vi "step_HAPS_Compressor_worksheet.vi"() -> ()   [LabVIEW 2020]
uses:
  <vilib>/AKKA/PROVEtech-RBS/PROVEtechRBS.lvlib
  <vilib>/AKKA/PROVEtech-RBS/SubVIs/Write (Signals Single-point).vi
  <vilib>/AKKA/PROVEtech-RBS/SubVIs/Read (Signals Single-point).vi
panel:
  out "receive unit":string[](array[string])
  out "pass":bool
  out "Array out":string[](array[string])
  out "receive signals":string[](array[string])
  out "sgl array":dbl[](array[numeric])
  out "send unit":string[](array[string])
  out "send values":string[](array[string])
  out "send signals":string[](array[string])
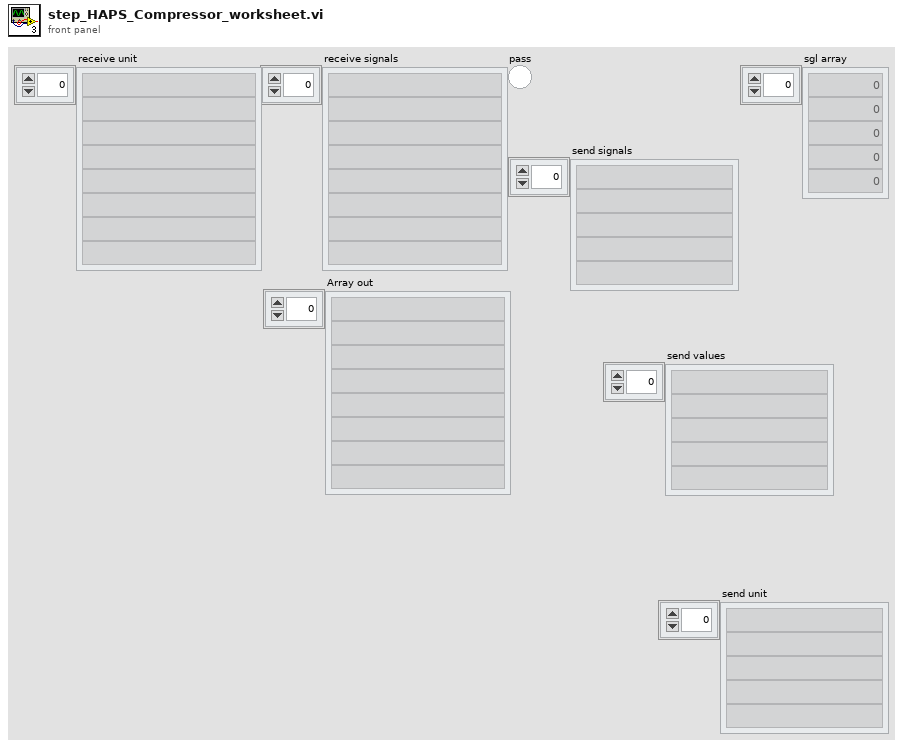
[diagram p1: front panel]
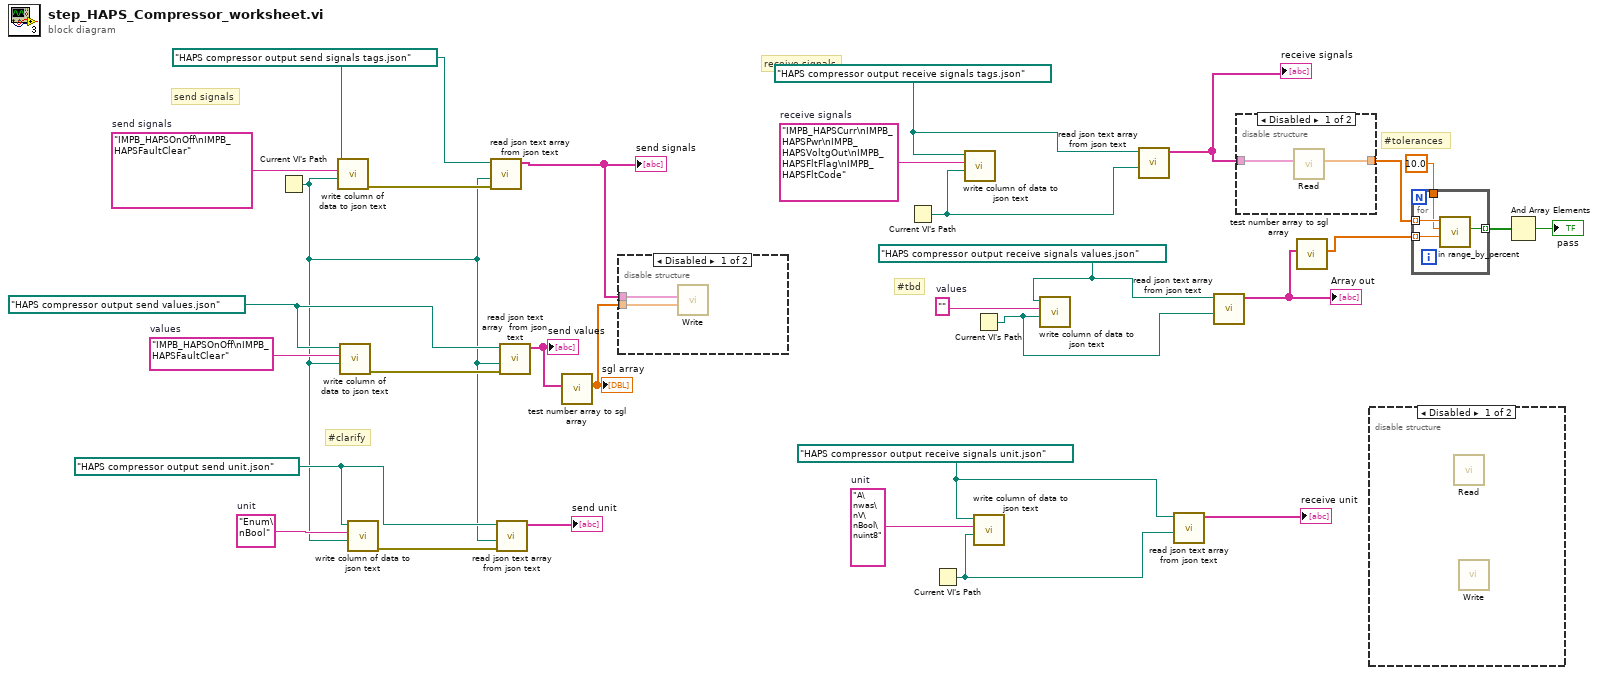
[diagram p0: block diagram]
diagram:
  w3 = path "HAPS compressor output receive signals unit.json" ("name or relative path")
  w13 = path "HAPS compressor output receive signals values.json" ("name or relative path")
  w23 = path "HAPS compressor output send unit.json" ("name or relative path")
  w26 = path "HAPS compressor output send values.json" ("name or relative path")
  w16 = path "HAPS compressor output receive signals tags.json" ("name or relative path")
  w29 = path "HAPS compressor output send signals tags.json" ("name or relative path")
  w14 = ""  # values
  w1 = "A\nwas\nV\nBool\nuint8"  # unit
  w17 = "IMPB_HAPSCurr\nIMPB_HAPSPwr\nIMPB_HAPSVoltgOut\nIMPB_HAPSFltFlag\nIMPB_HAPSFltCode"  # receive signals
  w24 = "Enum\nBool"  # unit
  w27 = "IMPB_HAPSOnOff\nIMPB_HAPSFaultClear"  # values
  w31 = "IMPB_HAPSOnOff\nIMPB_HAPSFaultClear"  # send signals
  # "#tolerances"
  # "#clarify"
  # "#tbd"
  # "receive signals"
  # "send signals"
  n1 = Current VI's Path() -> (path=w21:path)
  n2 = call "write column of data to json text.vi"("this vi path"=w21, "column of data"=w31, "file name"=w29) -> ("error out"=w30:errorcluster)  [unwired: 8 in]
  n3 = call "write column of data to json text.vi"("this vi path"=w21, "column of data"=w27, "file name"=w26) -> ("error out"=w28:errorcluster)  [unwired: 8 in]
  n4 = call "write column of data to json text.vi"("this vi path"=w21, "column of data"=w24, "file name"=w23) -> ("error out"=w25:errorcluster)  [unwired: 8 in]
  n5 = call "read json text array  from json text.vi"("error in (no error)"=w30, "this vis path"=w21, "file name"=w29) -> ("Array out"=w19:string[])  [unwired: 7 in, 1 out]
  "send signals" <- w19
  n6 = call "read json text array  from json text.vi"("error in (no error)"=w25, "this vis path"=w21, "file name"=w23) -> ("Array out"=→"send unit":string[])  [unwired: 7 in, 1 out]
  n7 = call "read json text array  from json text.vi"("error in (no error)"=w28, "this vis path"=w21, "file name"=w26) -> ("Array out"=w20:string[])  [unwired: 7 in, 1 out]
  "send values" <- w20
  n8 = call "test number array to sgl array.vi"("send values"=w20) -> ("sgl array"=w18:dbl[])  [unwired: 10 in]
  "sgl array" <- w18
  n9 = disable-structure shown="Disabled" {
    disable-tunnel: w19 -> [w33 _]
    disable-tunnel: w18 -> [w32 _]
    frame Disabled {
      n10 = call-poly <vilib>:"Write.vi"("values"=w32, "signals"=w33) -> ()  [unwired: 8 in, 2 out]
    }
    frame Enabled {
    }
  }
  n11 = Current VI's Path() -> (path=w15:path)
  n12 = Current VI's Path() -> (path=w4:path)
  n13 = call "write column of data to json text.vi"("this vi path"=w15, "column of data"=w17, "file name"=w16) -> ()  [unwired: 8 in, 1 out]
  n14 = Current VI's Path() -> (path=w12:path)
  n15 = call "write column of data to json text.vi"("this vi path"=w4, "column of data"=w1, "file name"=w3) -> ()  [unwired: 8 in, 1 out]
  n16 = call "write column of data to json text.vi"("this vi path"=w12, "column of data"=w14, "file name"=w13) -> ()  [unwired: 8 in, 1 out]
  n17 = call "read json text array  from json text.vi"("this vis path"=w15, "file name"=w16) -> ("Array out"=w10:string[])  [unwired: 8 in, 1 out]
  "receive signals" <- w10
  n18 = call "read json text array  from json text.vi"("this vis path"=w4, "file name"=w3) -> ("Array out"=→"receive unit":string[])  [unwired: 8 in, 1 out]
  n19 = call "read json text array  from json text.vi"("this vis path"=w12, "file name"=w13) -> ("Array out"=w11:string[])  [unwired: 8 in, 1 out]
  "Array out" <- w11
  n20 = disable-structure shown="Disabled" {
    disable-tunnel: w10 -> [w35 _]
    disable-tunnel: [w34 _] -> w9
    frame Disabled {
      n21 = call-poly <vilib>:"Read.vi"("signals"=w35) -> ("values"=w34:dbl[])  [unwired: 8 in, 2 out]
    }
    frame Enabled {
    }
  }
  n22 = call "test number array to sgl array.vi"("send values"=w11) -> ("sgl array"=w8:dbl[])  [unwired: 10 in]
  n23 = disable-structure shown="Disabled" {
    frame Disabled {
      n24 = call-poly <vilib>:"Read.vi"() -> ()  [unwired: 9 in, 3 out]
      n25 = call-poly <vilib>:"Write.vi"() -> ()  [unwired: 10 in, 2 out]
    }
    frame Enabled {
    }
  }
  n26 = for {
    tunnel: w9 -> [w39] mode=indexing
    tunnel: w8 -> [w38] mode=indexing
    tunnel: 10.0 ("tol %") -> [w37]
    tunnel: [w36] -> w6 mode=indexing
    n27 = call "in range_by_percent.vi"("setpoint"=w38, "tol %"=w37, "x"=w39) -> ("In Range?"=w36:bool)  [unwired: 5 in, 3 out]
  }
  n28 = And Array Elements(Boolean array=w6) -> (logical AND=→"pass":bool)
